vi "Elapsed Timer.vi"(7 "Timer Control":T1, 8 "error in (no error)":errorcluster, 10 "Timeout (ms)":dbl) -> (0 "error out":errorcluster, 1 "Time Elapsed (ms)":dbl, 2 "Time Elapsed?":bool)   [LabVIEW 2010, in "Core SubVIs.lvlib"]
doc: "This VI will track a ms timer to determine when a user input amount of time (ms) has elapsed. Contains functions for reading elapsed time and resetting the timer."
uses:
  Core SubVIs.lvlib
  Controls/TYPE - Timer Control.ctl
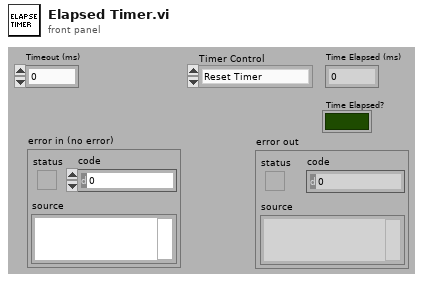
[diagram p1: front panel]
types:
  T1 = typedef "Core SubVIs.lvlib/TYPE - Timer Control.ctl" = enum16{"Reset Timer", "Read Timer"}
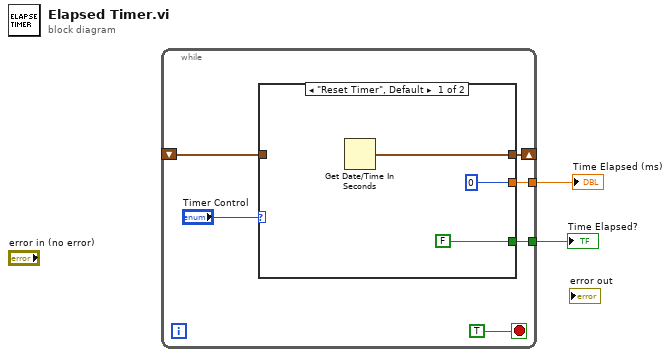
[diagram p0: block diagram]
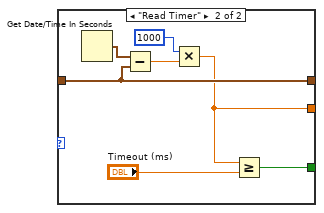
[diagram p2: hidden frame]
diagram:
  n1 = while {
    shift-right: [w6] -> _
    shift-left: _ -> [w4]
    tunnel: [w5] -> w2
    tunnel: [w3] -> w1
    stop <- TRUE stop-if-true
    n2 = case shown="\"Reset Timer\", Default" "Timer Control" {
      tunnel: [w9 w18] -> w6
      tunnel: [FALSE ("Time Elapsed?") w17] -> w5
      tunnel: w4 -> [_ w18]
      tunnel: [u32 0 w12] -> w3
      frame "Reset Timer", Default {
        n3 = Get Date/Time In Seconds() -> (seconds since 1Jan1904=w9:timestamp)
      }
      frame "Read Timer" {
        n4 = Get Date/Time In Seconds() -> (seconds since 1Jan1904=w16:timestamp)
        n5 = Subtract(x=w16, y=w18) -> (x-y=w14:dbl)
        n6 = Multiply(x=1000, y=w14) -> (x*y=w12:dbl)
        n7 = Greater Or Equal?(x=w12, y="Timeout (ms)") -> (x >= y?=w17:bool)
      }
    }
  }
  "Time Elapsed?" <- w2
  "Time Elapsed (ms)" <- w1
